vi "Address Space Size.vi"(2 "AddressSpace":refnum<class "AddressSpace.lvclass">) -> (6 "size":u32)   [LabVIEW 2017, in "ActiveFrontEnd.lvlib" / "AddressSpace.lvclass"]
uses:
  AddressSpace.lvclass
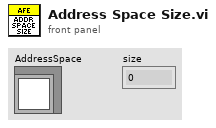
[diagram p1: front panel]
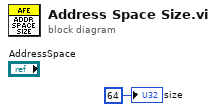
[diagram p0: block diagram]
diagram:
  "size" <- u32 64 ("size")
